vi "GetTriggerCount.vi"(8 "Error In":errorcluster, 11 "Keithley 6485 In":refnum<visa-resource-name>) -> (0 "Error Out":errorcluster, 2 "Count (1-3000)":u16, 3 "Keithley 6485 Out":refnum<visa-resource-name>)   [LabVIEW 2012, in "Keithley-6485.lvlib"]
uses:
  Keithley-6485.lvlib
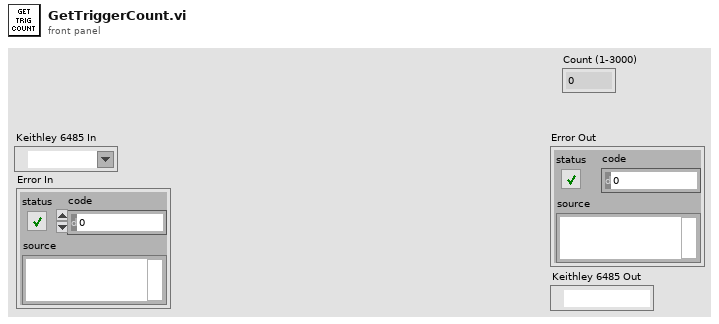
[diagram p1: front panel]
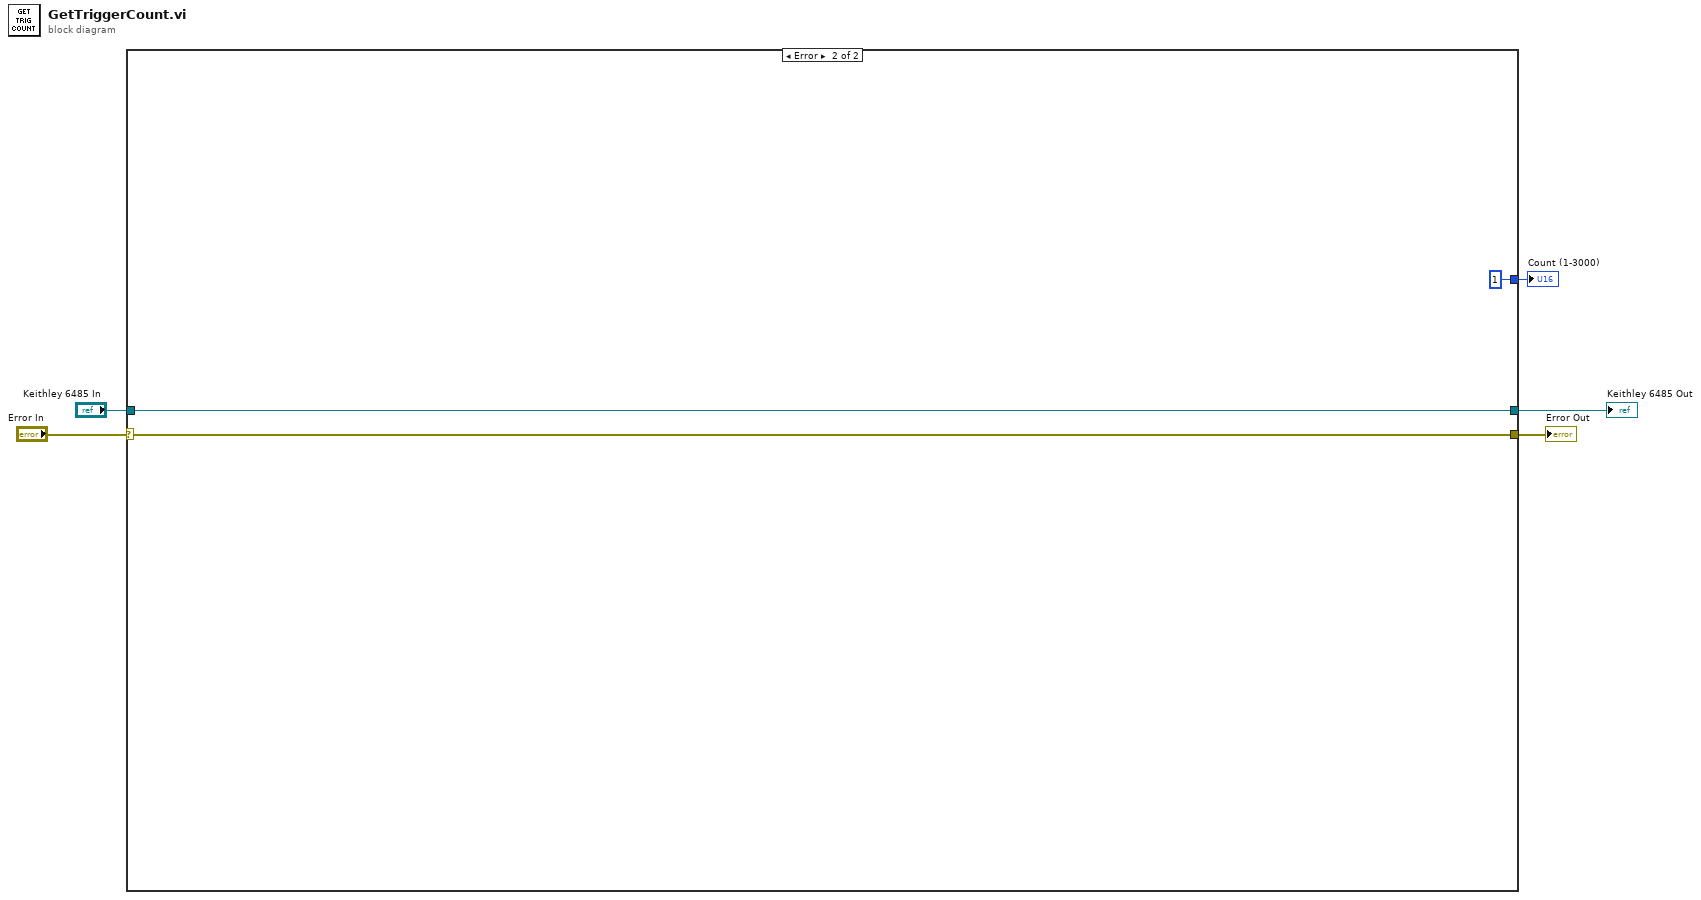
[diagram p0: block diagram]
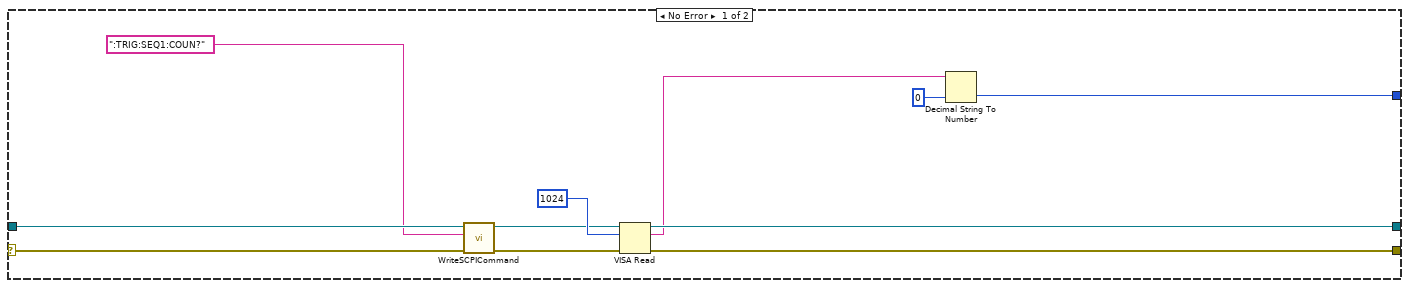
[diagram p2: hidden frame]
diagram:
  n1 = case shown="Error" "Error In" {
    selector: "Error In" -> [w11 w18]
    tunnel: "Keithley 6485 In" -> [w10 w19]
    tunnel: [w16 w18] -> w3
    tunnel: [w15 w19] -> w2
    tunnel: [w9 u16 1] -> w1
    frame No Error {
      n2 = call "WriteSCPICommand.vi"("Error In"=w11, "SCPI Command"=":TRIG:SEQ1:COUN?" ("string"), "Keithley 6482 In"=w10) -> ("Error Out"=w12:errorcluster, "Keithley 6482 Out"=w13:refnum<visa-resource-name>)  [unwired: 7 in]
      n3 = VISA Read(VISA resource name=w13, byte count=u32 1024, error in (no error)=w12) -> (VISA resource name out=w15:refnum<visa-resource-name>, read buffer=w7:string, error out=w16:errorcluster)  [unwired: 1 out]
      n4 = Decimal String To Number(string=w7, default (0L)=u16 0) -> (number=w9:u16)  [unwired: 1 in, 1 out]
    }
    frame Error {
    }
  }
  "Error Out" <- w3
  "Keithley 6485 Out" <- w2
  "Count (1-3000)" <- w1
